vi "struct_abs_act_g_Txv1v2.vi"(0 "Reference working pair (Input)":i64, 1 "Molar volume of second component in m3/mol (Input)":dbl, 5 "Temperature in K (Input)":dbl, 7 "Mole fraction in liquid phase in mol/mol (Input)":dbl, 9 "Molar volume of first component in m3/mol (Input)":dbl, 11 "Error (Input)":errorcluster) -> (4 "Activity coefficient of first component (Output)":dbl, 15 "Error (Output)":errorcluster)   [LabVIEW 2017]
doc: "abs_act_g_Txv1v2:\n * -----------------\n *\n * Calculates activity coefficient of first component depending on temperature\n * T_K in K, mole fraction in liquid phase x_molmol in mol/mol, molar volume of\n * first component in m³/mol, and molar volume of second component in m³/mol.\n *\n * Parameters:\n * -----------\n * double T_K:\n * Equilibrium temperature in K.\n * double x_molmol:\n * Equilibrium mole fraction in liquid phase in mol/mol.\n * double v1_m3mol:\n * Equilibrium molar volume of first component in m³/mol.\n * double v2_m3mol:\n * Equilibrium molar volume of second component in m³/mol.\n * struct *WorkingPair:\n * Pointer of WorkingPair-struct.\n *\n * Returns:\n * --------\n * double:\n * Activity coefficient of first component.\n *\n * Remarks:\n * --------\n * This function is only valid for isotherm models based on activity\n * coefficients.\n * Molar volumes may are not required and ignored. When molar volumes are\n * required, function uses molar volumes stored in JSON file when input\n * v1_m3mol or v2_m3mol is -1. Otherwise, function uses molar volumes given by\n * inputs.\n *\n * History:\n * --------\n * 07/14/2021, by Jannik Driesel (supervised by Mirko Engelpracht):\n * First implementation."
uses:
  data/win32bit/libsorpPropLib.dll
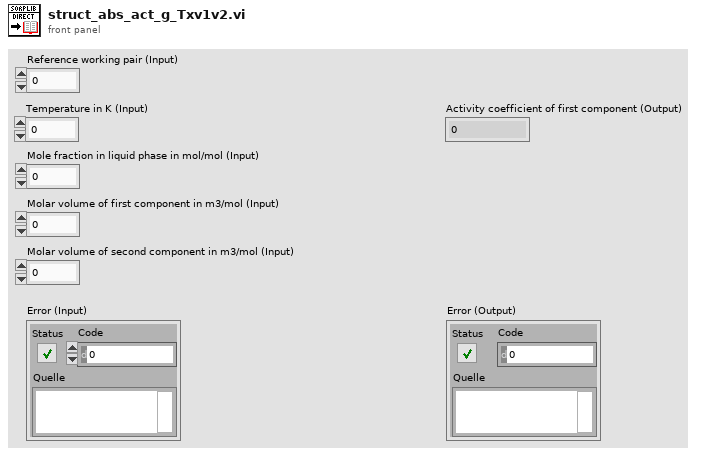
[diagram p1: front panel]
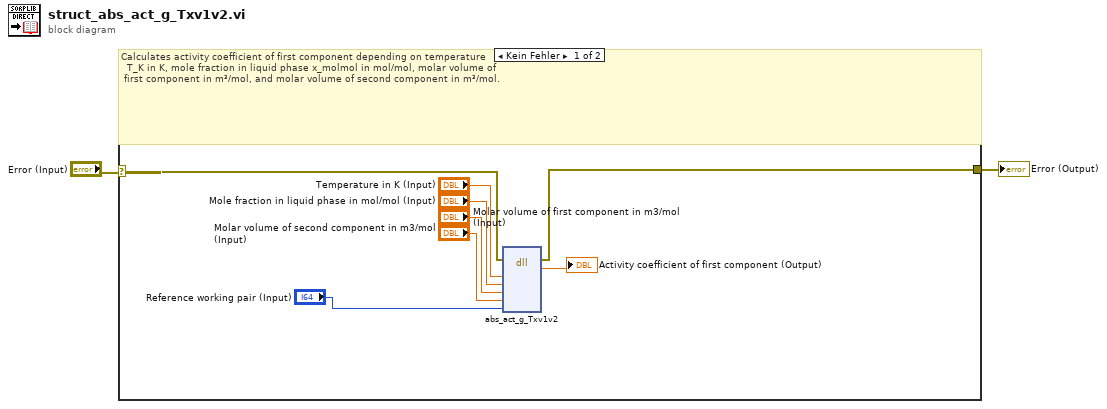
[diagram p0: block diagram]
diagram:
  n1 = case shown="Kein Fehler" "Error (Input)" {
    selector: "Error (Input)" -> [w10 w11]
    tunnel: [w9 w11] -> w2
    frame No Error {
      # "Calculates activity coefficient of first component depending on temperature\n  T_K in K, mole fraction in liquid phase x_molmol in mol/mol, molar volume of\n first component in m³/mol, and molar volume of second component in m³/mol."
      n2 = dll-call lib="D:/Driesel/SorpLibLocal/LabVIEW_wrapper/data/win32bit/libsorpPropLib.dll" fn="abs_act_g_Txv1v2"(error in=w10, "T_K"="Temperature in K (Input)", "x_molmol"="Mole fraction in liquid phase in mol/mol (Input)", "v1_m3mol"="Molar volume of first component in m3/mol (Input)", "v2_m3mol"="Molar volume of second component in m3/mol (Input)", "workingPair"="Reference working pair (Input)") -> (error out=w9:errorcluster, "g"=→"Activity coefficient of first component (Output)":dbl)  [unwired: 7 in, 1 out]
    }
    frame Error {
      # "Error - No calculations"
    }
  }
  "Error (Output)" <- w2
